vi "To String.vi"(7 "enable LabVIEW extensions? (T)":bool=TRUE, 8 "error in (no error)":errorcluster, 11 "JSON Helper in":refnum<class "JSON Value.lvclass">) -> (0 "error out":errorcluster, 3 "String":string)   [LabVIEW 2016, in "JSON Value.lvclass"]
uses:
  JSON Value.lvclass
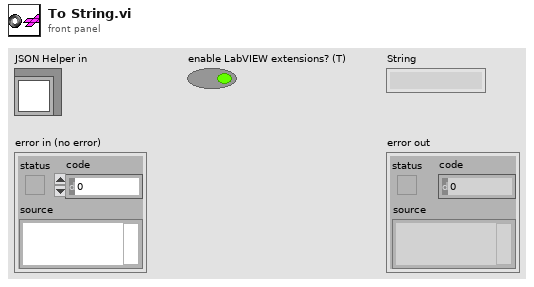
[diagram p1: front panel]
types:
  T1 = typedef "JSON Value.lvclass/JSON Types.ctl" = enum16{"String", "Numeric", "Boolean", "NULL", "Object", "Array"}
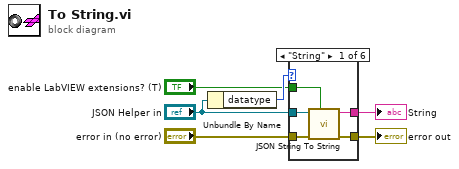
[diagram p0: block diagram]
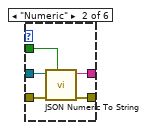
[diagram p2: hidden frame]
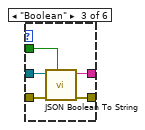
[diagram p3: hidden frame]
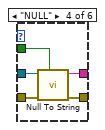
[diagram p4: hidden frame]
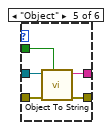
[diagram p5: hidden frame]
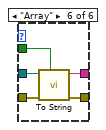
[diagram p6: hidden frame]
diagram:
  n1 = Unbundle By Name("JSON Helper in") -> ("datatype"=w6:T1)
  n2 = case shown="\"String\"" w6 {
    tunnel: [w11 w16 w21 w26 w31 w36] -> w5
    tunnel: [w10 w15 w20 w25 w30 w35] -> w4
    tunnel: "enable LabVIEW extensions? (T)" -> [w9 w14 w19 w24 w29 w34]
    tunnel: "error in (no error)" -> [w8 w13 w18 w23 w28 w33]
    tunnel: "JSON Helper in" -> [w7 w12 w17 w22 w27 w32]
    frame "String" {
      n3 = call "JSON String To String.vi"("enable LabVIEW extensions? (T)"=w9, "error in (no error)"=w8, "JSON String in"=w7) -> ("error out"=w11:errorcluster, "String"=w10:string)  [unwired: 7 in]
    }
    frame "Numeric" {
      n4 = call "JSON Numeric To String.vi"("enable LabVIEW extensions? (T)"=w14, "error in (no error)"=w13, "JSON Numeric in"=w12) -> ("error out"=w16:errorcluster, "String"=w15:string)  [unwired: 7 in]
    }
    frame "Boolean" {
      n5 = call "JSON Boolean To String.vi"("enable LabVIEW extensions? (T)"=w19, "error in (no error)"=w18, "JSON Boolean in"=w17) -> ("error out"=w21:errorcluster, "String"=w20:string)  [unwired: 7 in]
    }
    frame "NULL" {
      n6 = call "Null To String.vi"("enable LabVIEW extensions? (T)"=w24, "error in (no error)"=w23, "JSON Datatype in"=w22) -> ("error out"=w26:errorcluster, "String"=w25:string)  [unwired: 7 in]
    }
    frame "Object" {
      n7 = call "Object To String.vi"("enable LabVIEW extensions? (T)"=w29, "error in (no error)"=w28, "JSON Object in"=w27) -> ("error out"=w31:errorcluster, "String"=w30:string)  [unwired: 7 in]
    }
    frame "Array" {
      n8 = call "To String.vi"("enable LabVIEW extensions? (T)"=w34, "error in (no error)"=w33, "JSON Helper in"=w32) -> ("error out"=w36:errorcluster, "String"=w35:string)  [unwired: 7 in]
    }
  }
  "error out" <- w5
  "String" <- w4
